vi "Core - Exported Command.vi"(0 "LVx Command in":refnum<class "LVx.lvclass">, 5 "Session ID":string, 11 "error in (no error)":errorcluster, 13 "Init (F)":bool) -> (4 "LVx Command out":refnum<class "LVx.lvclass">, 6 "LVx Core Event":refnum<user-event>, 15 "error out":errorcluster)   [LabVIEW 2011, in "LVx.lvlib"]
uses:
  LVx.lvlib
  LVx.lvclass
panel:
  out "NaN/Path/Refnum?":bool
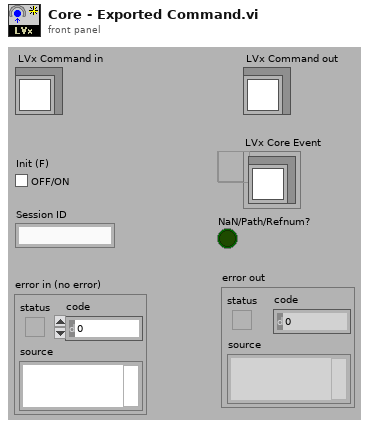
[diagram p1: front panel]
types:
  T1 = typedef "LVx.lvlib/LVx.lvclass/Typedef - LVx Response Notifier.ctl" = refnum<notifier>
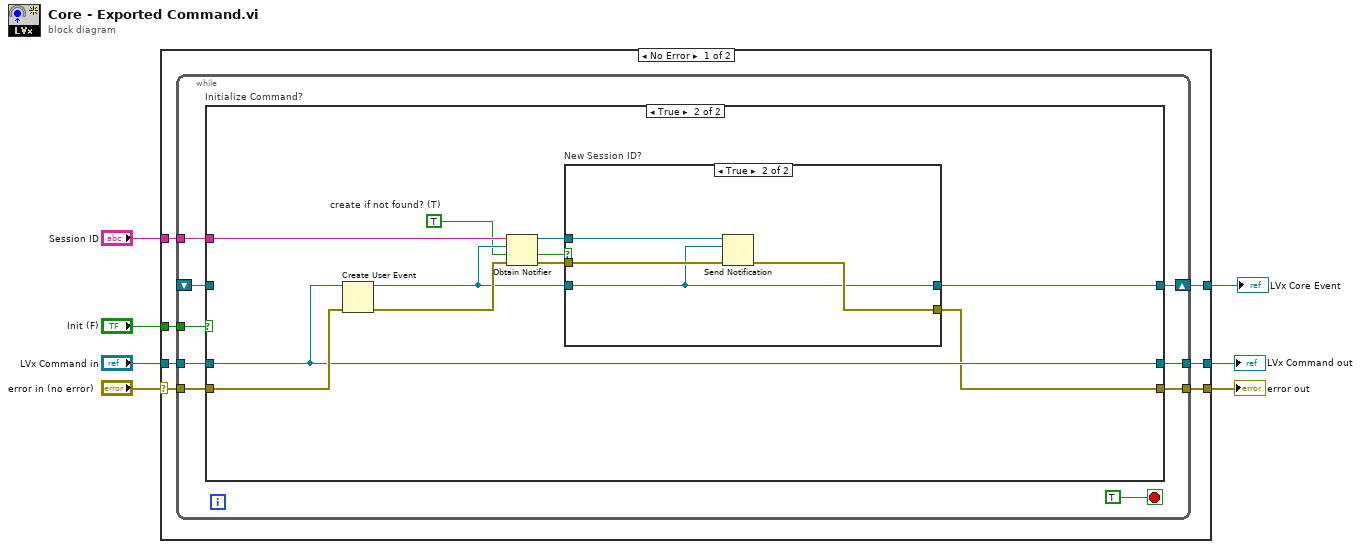
[diagram p0: block diagram]
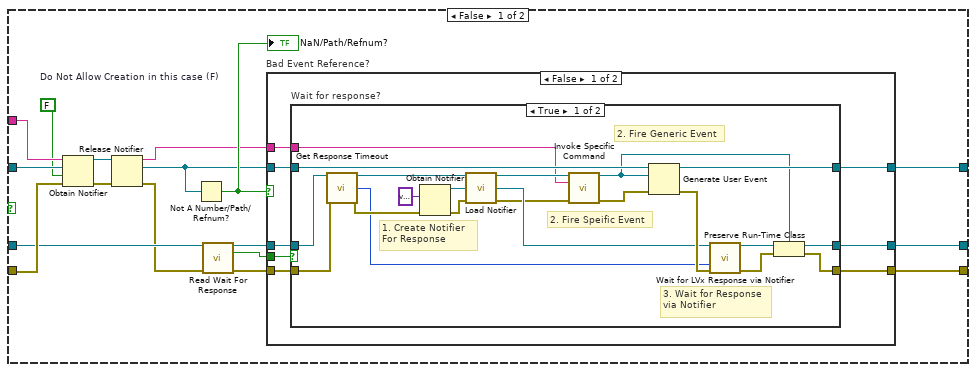
[diagram p2: hidden frame]
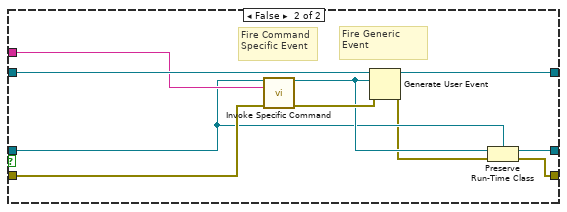
[diagram p3: hidden frame]
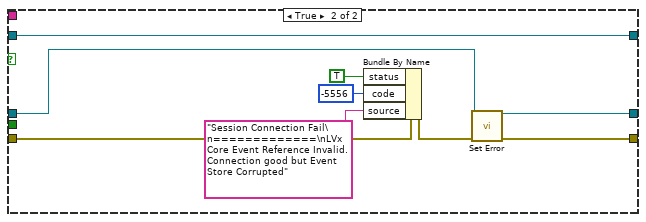
[diagram p4: hidden frame]
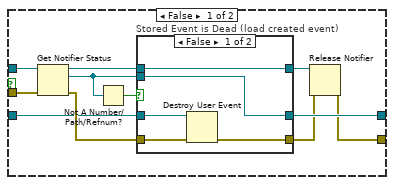
[diagram p5: hidden frame]
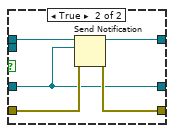
[diagram p6: hidden frame]
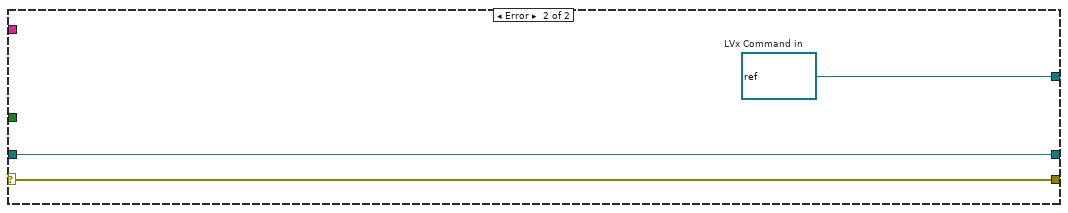
[diagram p7: hidden frame]
diagram:
  n1 = case shown="No Error" "error in (no error)" {
    selector: "error in (no error)" -> [w8 w127]
    tunnel: [w14 w127] -> w7
    tunnel: "LVx Command in" -> [w13 w126]
    tunnel: [w12 w126] -> w1
    tunnel: "Init (F)" -> [w11 _]
    tunnel: "Session ID" -> [w10 _]
    tunnel: [w9 w125] -> w4
    frame No Error {
      n2 = while {
        tunnel: [w23] -> w14
        tunnel: w8 -> [w18]
        tunnel: [w21] -> w12
        tunnel: w13 -> [w20]
        tunnel: w11 -> [w17]
        tunnel: w10 -> [w16]
        shift-right: [w19] -> w9
        shift-left: _ -> [w15]
        stop <- TRUE stop-if-true
        n3 = case "Initialize Command?" shown="True" w17 {
          tunnel: [w38 w89] -> w23
          tunnel: w18 -> [w30 w97]
          tunnel: [w39 w90] -> w21
          tunnel: w20 -> [w29 w90]
          tunnel: [w40 w92] -> w19
          tunnel: w16 -> [w32 w96]
          tunnel: w15 -> [w36 _]
          frame False {
            w31 = FALSE  # Do Not Allow Creation in this case (F)
            n4 = Obtain Notifier(name (unnamed)=w32, notification data type=w36, create if not found? (T)=w31, error in (no error)=w30) -> (notifier out=w27:refnum<notifier>, error out=w26:errorcluster)  [unwired: 1 out]
            n5 = Release Notifier(notifier=w27, error in (no error)=w26) -> (notifier name=w25:string, last notification=w24:refnum<user-event>, error out=w28:errorcluster)  [unwired: 1 in]
            n6 = Not A Number/Path/Refnum?(number/path/refnum=w24) -> (NaN/Path/Refnum?=w33:bool)
            "NaN/Path/Refnum?" <- w33
            n7 = call-dynamic "Read Wait For Response.vi"("LVx.lvclass in"=w29, "error in (no error)"=w28) -> ("LVx.lvclass out"=w34:refnum<class "LVx.lvclass">, "Wait For Response?"=w35:bool, "error out"=w37:errorcluster)  [unwired: 11 in]
            n8 = case "Bad Event Reference?" shown="False" w33 {
              tunnel: [w48 w88] -> w40
              tunnel: [w47 w80] -> w39
              tunnel: [w46 w87] -> w38
              tunnel: w34 -> [w45 w81]
              tunnel: w37 -> [w44 w86]
              tunnel: w35 -> [w43 _]
              tunnel: w24 -> [w42 w88]
              tunnel: w25 -> [w41 _]
              frame False {
                n9 = case "Wait for response?" shown="True" w43 {
                  tunnel: [w69 w79] -> w48
                  tunnel: [w64 w73] -> w47
                  tunnel: [w62 w70] -> w46
                  tunnel: w42 -> [w67 w78]
                  tunnel: w45 -> [w60 w72]
                  tunnel: w44 -> [w61 w77]
                  tunnel: w41 -> [w49 w75]
                  frame True {
                    # "2. Fire Generic Event"
                    # "3. Wait for Response\nvia Notifier"
                    # "1. Create Notifier  For Response"
                    # "2. Fire Speific Event"
                    n10 = call-dynamic "Get Response Timeout.vi"("LVx In"=w60, "error in (no error)"=w61) -> ("LVx Out"=w55:refnum<class "LVx.lvclass">, "timeout in ms (-1:never)"=w56:i32, "error out"=w59:errorcluster)  [unwired: 11 in]
                    n11 = Obtain Notifier(notification data type=variant ("element data type"), error in (no error)=w59) -> (notifier out=w57:refnum<notifier>, error out=w54:errorcluster)  [unwired: 1 in, 2 out]
                    n12 = call "Load Notifier.vi"("LVx.lvlib:LVx.lvclass"=w55, "GUI Response Notifier"=w57, "error in (no error)"=w54) -> ("LVx.lvclass out"=w51:refnum<class "LVx.lvclass">, "GUI Response Notifier"=w58:T1, "error out"=w53:errorcluster)  [unwired: 1 in, 9 out]
                    n13 = call "Invoke Specific Command.vi"("LVx Command in"=w51, "Session ID"=w49, "error in (no error)"=w53) -> ("LVx Command out"=w50:refnum<class "LVx.lvclass">, "error out"=w52:errorcluster)  [unwired: 11 in]
                    n14 = Generate User Event(user event=w67, event data cluster=w50, error in=w52) -> (user event out=w69:refnum<user-event>, error out=w68:errorcluster)
                    n15 = call "Wait for LVx Response via Notifier.vi"("response notifier"=w58, "timeout in ms (10000)"=w56, "error in"=w68) -> ("data"=w65:refnum<class "LVx.lvclass">, "error out"=w63:errorcluster)  [unwired: 10 in, 1 out]
                    n16 = Preserve Run-Time Class(object in=w65, error in=w63, 2:w50) -> (object out=w64:refnum<class "LVx.lvclass">, error out=w62:errorcluster)
                  }
                  frame False {
                    # "Fire Command Specific Event"
                    # "Fire Generic Event"
                    n17 = call "Invoke Specific Command.vi"("LVx Command in"=w72, "Session ID"=w75, "error in (no error)"=w77) -> ("LVx Command out"=w74:refnum<class "LVx.lvclass">, "error out"=w76:errorcluster)  [unwired: 11 in]
                    n18 = Generate User Event(user event=w78, event data cluster=w74, error in=w76) -> (user event out=w79:refnum<user-event>, error out=w71:errorcluster)
                    n19 = Preserve Run-Time Class(object in=w74, error in=w71, 2:w72) -> (object out=w73:refnum<class "LVx.lvclass">, error out=w70:errorcluster)
                  }
                }
              }
              frame True {
                n20 = Bundle By Name(cluster=w86, "status"=TRUE, "code"=-5556, "source"="Session Connection Fail\n=============\nLVx Core Event Reference Invalid. Connection good but Event Store Corrupted") -> (w85:errorcluster)
                n21 = call "Set Error.vi"("LVx.lvlib:LVx.lvclass"=w81, "error in (no error)"=w85) -> ("LVx.lvlib:LVx.lvclass 2"=w80:refnum<class "LVx.lvclass">, "error out"=w87:errorcluster)  [unwired: 12 in]
              }
            }
          }
          frame True {
            w91 = TRUE  # create if not found? (T)
            n22 = Create User Event(user event datatype=w90, error in=w97) -> (user event=w94:refnum<user-event>, error out=w99:errorcluster)
            n23 = Obtain Notifier(name (unnamed)=w96, notification data type=w94, create if not found? (T)=w91, error in (no error)=w99) -> (notifier out=w95:refnum<notifier>, created new?=w93:bool, error out=w98:errorcluster)
            n24 = case "New Session ID?" shown="True" w93 {
              tunnel: w98 -> [w109 w124]
              tunnel: [w100 w123] -> w89
              tunnel: w95 -> [w108 w122]
              tunnel: w94 -> [w107 w121]
              tunnel: [w105 w121] -> w92
              frame False {
                n25 = Get Notifier Status(notifier=w108, error in (no error)=w109) -> (notifier out=w103:refnum<notifier>, current notification=w104:refnum<user-event>, error out=w110:errorcluster)  [unwired: 2 out]
                n26 = Not A Number/Path/Refnum?(number/path/refnum=w104) -> (NaN/Path/Refnum?=w106:bool)
                n27 = case "Stored Event is Dead (load created event)" shown="False" w106 {
                  tunnel: w110 -> [w115 w119]
                  tunnel: w107 -> [w114 w117]
                  tunnel: [w113 w118] -> w101
                  tunnel: [w112 w117] -> w105
                  tunnel: w104 -> [w112 _]
                  tunnel: w103 -> [w111 w120]
                  tunnel: [w111 w116] -> w102
                  frame False {
                    n28 = Destroy User Event(user event=w114, error in=w115) -> (error out=w113:errorcluster)
                  }
                  frame True {
                    n29 = Send Notification(notification=w117, notifier=w120, error in (no error)=w119) -> (notifier out=w116:refnum<notifier>, error out=w118:errorcluster)
                  }
                }
                n30 = Release Notifier(notifier=w102, error in (no error)=w101) -> (error out=w100:errorcluster)  [unwired: 1 in, 2 out]
              }
              frame True {
                n31 = Send Notification(notification=w121, notifier=w122, error in (no error)=w124) -> (error out=w123:errorcluster)  [unwired: 1 out]
              }
            }
          }
        }
      }
    }
    frame Error {
      w125 = refnum<user-event> refnum  # LVx Command in
    }
  }
  "error out" <- w7
  "LVx Command out" <- w1
  "LVx Core Event" <- w4
